vi "Graph Color Legend.vi"(6 "Control Ref Queue":T5, 7 "Multiplot Representation In":T1, 8 "error in (no error)":errorcluster, 9 "Former Ignore States":bool, 11 "3D Pie.lvclass in":refnum<class "3D Pie.lvclass">) -> (0 "error out":errorcluster, 1 "Ignore the size change?":bool, 3 "3D Pie.lvclass out":refnum<class "3D Pie.lvclass">, 5 "Multiplot Representation Out":T1)   [LabVIEW 2017, in "3D Pie.lvclass"]
uses:
  <vilib>/Math Plots/3D Math Plots/3D Pie/3D Pie/3D Pie.lvclass
  e:/builds/penguin/labview/branches/2017/dev/dist/vi.lib/Math Plots/3D Math Plots/3D Plot/3D Plot/3D Plot.lvclass
  <vilib>/Math Plots/3D Math Plots/3D Plot/Action String/3DMathPlot Ctrl Act Queue.ctl
  <vilib>/Math Plots/3D Math Plots/3D Plot/Action String/3DMathPlot Ctrl Act Cluster.ctl
  <vilib>/Math Plots/3D Math Plots/3D Plot/Action String/3DMathPlot State Class.ctl
  <vilib>/Math Plots/3D Math Plots/3D Plot/3D Plot/Typedef/Multiplot Representation.ctl
  <vilib>/Math Plots/3D Math Plots/3D Plot/3D Plot/Typedef/Plot Representation.ctl
  <vilib>/Math Plots/3D Math Plots/3D Plot/3D Plot/Typedef/Range Clusters.ctl
  <vilib>/Math Plots/3D Math Plots/3D Plot/3D Plot/Typedef/Mesh Data.ctl
  <vilib>/Math Plots/3D Math Plots/3D Pie/3D Pie/3D Pie.lvclass/3D Pie.ctl
  <vilib>/Math Plots/3D Math Plots/3D Plot/3D Plot/3D Plot.lvclass
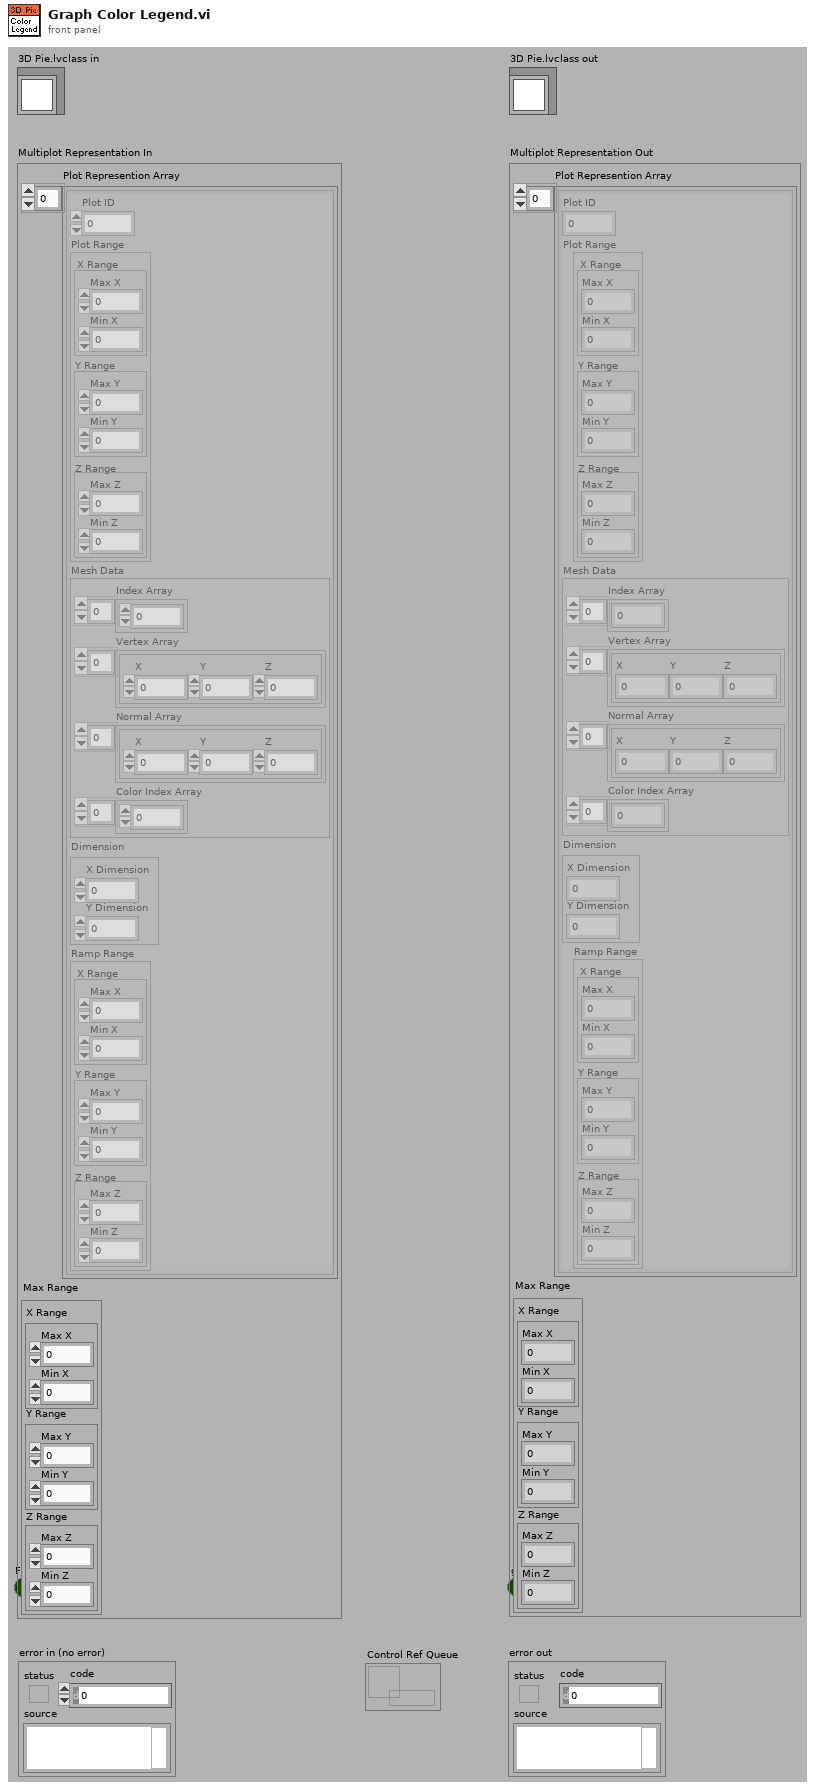
[diagram p1: front panel]
types:
  T1 = typedef "3D Plot.lvclass/Multiplot Representation.ctl" = cluster{"Plot Represention Array":T2[], "Max Range":T3}
  T2 = typedef "3D Plot.lvclass/Plot Representation.ctl" = cluster{"Plot ID":i32, "Plot Range":T3, "Mesh Data":T4, "Dimension":cluster{"X Dimension":i32, "Y Dimension":i32}, "Ramp Range":T3}
  T3 = typedef "3D Plot.lvclass/Range Clusters.ctl" = cluster{"X Range":cluster{"Max X":sgl, "Min X":sgl}, "Y Range":cluster{"Max Y":sgl, "Min Y":sgl}, "Z Range":cluster{"Max Z":sgl, "Min Z":sgl}}
  T4 = typedef "3D Plot.lvclass/Mesh Data.ctl" = cluster{"Index Array":u32[], "Vertex Array":cluster{"X":sgl, "Y":sgl, "Z":sgl}[], "Normal Array":cluster{"X":sgl, "Y":sgl, "Z":sgl}[], "Color Index Array":i32[]}
  T5 = typedef "3DMathPlot Ctrl Act Queue.ctl" = refnum<queue>
  T6 = typedef "3D Pie.lvclass/3D Pie Property Array.ctl" = T7[]
  T7 = typedef "3D Pie.lvclass/3D Pie Property.ctl" = cluster{"General Property":cluster{"Plot Name":string, "Coordinate System":enum16{"Cartesian", "Cylindrical", "Spherical"}, "Opacity":sgl}, "Projection Property":cluster{"Draw XY":bool, "Draw YZ":bool, "Draw XZ":bool}, "Plot Property":cluster{"Line Style":T8, "Line Width":sgl, "Line Color":u32, "Antialiasing":bool}, "Pie Property":cluster{"Pie Height":sgl, "Pie Center":cluster{"X":sgl, "Y":sgl, "Z":sgl}, "Label Mode":enum16{"None", "Show Percentage", "Show String"}, "Label Size":u16, "Label Color":u32, "Color Pair Array":cluster{"Color":u32, "String":string}[], "Slice Offset?":bool}}
  T8 = typedef "3D Plot.lvclass/Line Type.ctl" = enum16{"None", "Solid", "Dash", "Dot", "Dash Dot"}
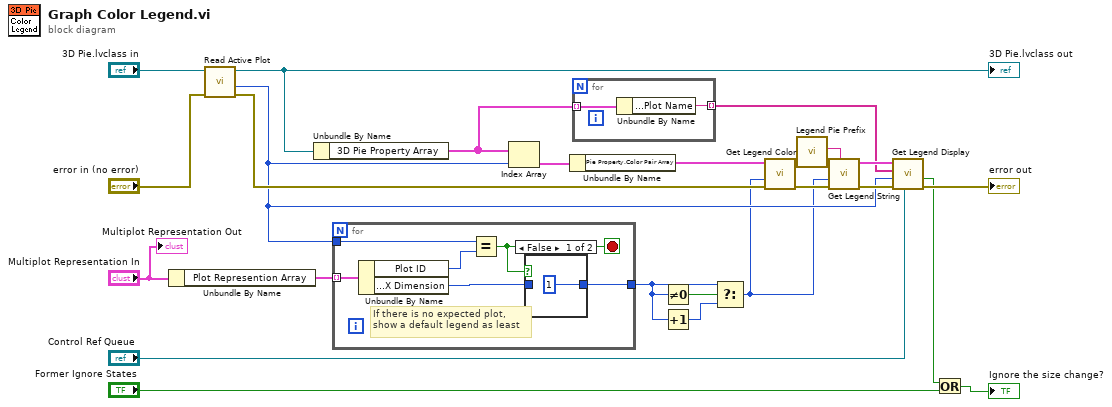
[diagram p0: block diagram]
diagram:
  n1 = Unbundle By Name("Multiplot Representation In") -> ("Plot Represention Array"=w5:T2[])
  n2 = call <vilib>:"Read Active Plot.vi"("error in (no error)"="error in (no error)", "3D Plot.lvclass in"="3D Pie.lvclass in") -> ("error out"=w9:errorcluster, "Active Plot"=w7:i32, "3D Plot.lvclass out"=w22:refnum<class "3D Pie.lvclass">)  [unwired: 7 out]
  "3D Pie.lvclass out" <- w22
  n3 = Unbundle By Name(w22) -> ("3D Pie Property Array"=w8:T6)
  n4 = for {
    tunnel: w5 -> [w29] mode=indexing
    tunnel: w7 -> [w27]
    tunnel: [w25] -> w2
    stop <- w26 stop-if-true
    # "If there is no expected plot,\nshow a default legend as least"
    n5 = Unbundle By Name(w29) -> ("Plot ID"=w28:i32, "Dimension.X Dimension"=w24:i32)
    n6 = Equal?(x=w27, y=w28) -> (x = y?=w26:bool)
    n7 = case shown="False" w26 {
      tunnel: [1 ("X Dimension") w31] -> w25
      tunnel: w24 -> [_ w31]
      frame False {
      }
      frame True {
      }
    }
  }
  n8 = Index Array(array=w8, index=w7) -> (element=w11:T7)
  n9 = Unbundle By Name(w11) -> ("Pie Property.Color Pair Array"=w12:cluster{"Color":u32, "String":string}[])
  n10 = for {
    tunnel: w8 -> [w33] mode=indexing
    tunnel: [w32] -> w10 mode=indexing
    n11 = Unbundle By Name(w33) -> ("General Property.Plot Name"=w32:string)
  }
  n12 = Not Equal To 0?(x=w2) -> (x != 0?=w4:bool)
  n13 = Increment(x=w2) -> (x+1=w3:i32)
  n14 = Select(t=w2, s=w4, f=w3) -> (s? t:f=w1:i32)
  n15 = call <vilib>:"Get Legend Color.vi"("Pair Array Length"=w1, "Color Pair Array In"=w12) -> ("Color Pair Array Out"=w14:cluster{"Color":u32, "String":string}[])  [unwired: 9 out]
  n16 = call <vilib>:"Legend Pie Prefix.vi"() -> ("Prefix Out"=w6:string)  [unwired: 11 out]
  n17 = call <vilib>:"Get Legend String.vi"("Initial String"=w6, "Pair Array Length"=w1, "Color Pair Array In"=w14) -> ("Color Pair Array Out"=w13:cluster{"Color":u32, "String":string}[])  [unwired: 8 out]
  n18 = call <vilib>:"Get Legend Display.vi"("Control Ref Queue"="Control Ref Queue", "error in (no error)"=w9, "Active Plot"=w7, "Plot Name"=w10, "Color Pair Array"=w13) -> ("error out"=→"error out":errorcluster, "Ignore the size change?"=w15:bool)  [unwired: 5 out]
  n19 = Or(x=w15, y="Former Ignore States") -> (x .or. y?=→"Ignore the size change?":bool)
  "Multiplot Representation Out" <- "Multiplot Representation In"
